vi "Connection_working.vi"() -> ()   [LabVIEW 2015]
panel:
  out "Is minima found?":bool
  out "sign bits:\n191 for -1\n 63   for  1":u8
  in  "Stop":bool
  out "binary data in ASCII":string
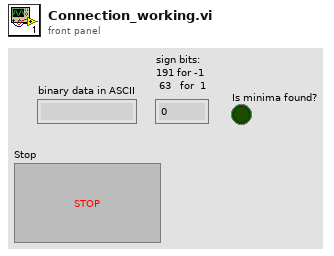
[diagram p1: front panel]
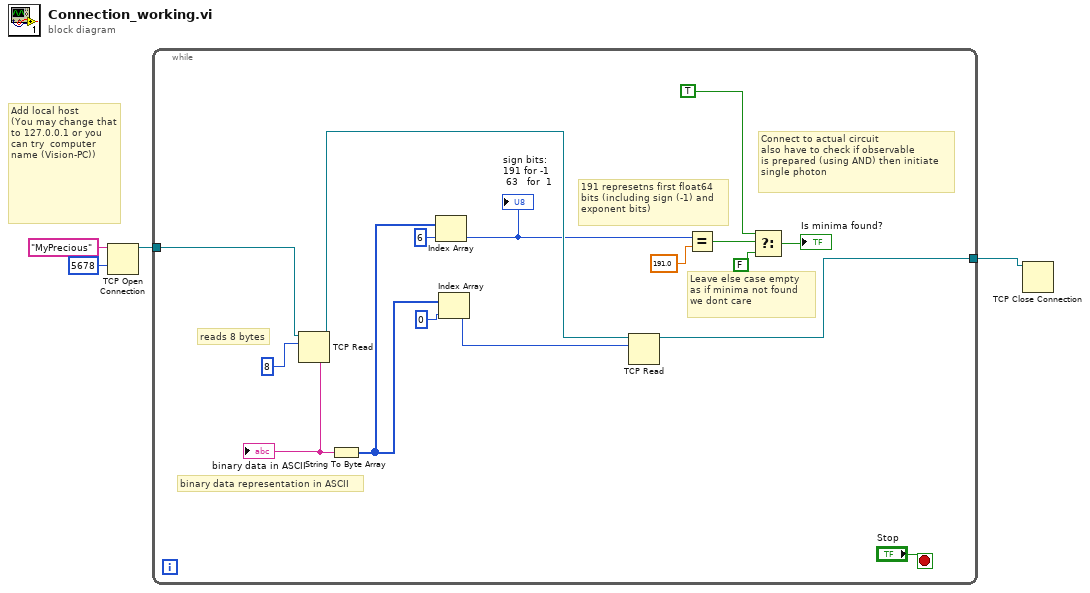
[diagram p0: block diagram]
diagram:
  # "Add local host\n(You may change that to 127.0.0.1 or you can try  computer name (Vision-PC))"
  n1 = TCP Open Connection(address="MyPrecious", remote port or service name=u16 5678) -> (connection ID=w1:refnum<k5>)  [unwired: 3 in, 1 out]
  n2 = while {
    tunnel: [w18] -> w4
    tunnel: w1 -> [w17]
    stop <- "Stop" stop-if-true
    # "binary data representation in ASCII"
    # "reads 8 bytes"
    # "Leave else case empty\nas if minima not found \nwe dont care"
    # "Connect to actual circuit\nalso have to check if observable \nis prepared (using AND) then initiate\nsingle photon"
    # "191 represetns first float64\nbits (including sign (-1) and\nexponent bits)"
    n3 = TCP Read(connection ID=w17, bytes to read=8) -> (connection ID out=w20:refnum<k5>, data out=w15:string)  [unwired: 3 in, 1 out]
    "binary data in ASCII" <- w15
    n4 = String To Byte Array(string=w15) -> (unsigned byte array=w11:u8[])
    n5 = Index Array(array=w11, index=6) -> (element=w9:u8)
    "sign bits:\n191 for -1\n 63   for  1" <- w9
    n6 = Index Array(array=w11, index=0) -> (element=w14:u8)
    n7 = TCP Read(connection ID=w20, bytes to read=w14) -> (connection ID out=w18:refnum<k5>)  [unwired: 3 in, 2 out]
    n8 = Equal?(x=w9, y=191.0) -> (x = y?=w8:bool)
    n9 = Select(t=TRUE, s=w8, f=FALSE) -> (s? t:f=→"Is minima found?":bool)
  }
  n10 = TCP Close Connection(connection ID=w4) -> ()  [unwired: 2 in, 2 out]
